vi "6060_read_all_I-O.vi"(1 "Address (Main, Sub reqd.)":T1, 2 "Channel Name":string) -> (3 "Comment":string, 4 "Input chs.":u8 format="%04b", 5 "Single Input Channel":i16)   [LabVIEW 2010]
uses:
  ADAM Client/Sub VIs/ADAM Controls/Address.ctl
panel:
  out "Output chs.":u8 format="%04b"
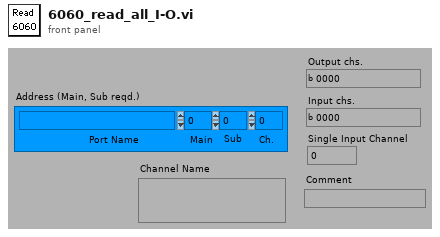
[diagram p1: front panel]
types:
  T1 = typedef "Address.ctl" = cluster{"Main":i32, "Ch.":i32, "Sub":i32, "Port Name":string}
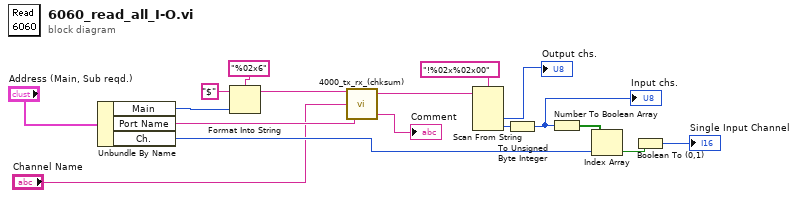
[diagram p0: block diagram]
diagram:
  n1 = Unbundle By Name("Address (Main, Sub reqd.)") -> ("Main"=w17:i32, "Port Name"=w10:string, "Ch."=w7:i32)
  n2 = Format Into String(format string="%02x6", initial string="$", w17) -> (resulting string=w14:string)  [unwired: 1 in, 1 out]
  n3 = call "4000_tx_rx_(chksum).vi"("Port Name"=w10, "Channel Name"="Channel Name", "Write String"=w14) -> ("Comment out"=→"Comment":string, "Read"=w9:string)  [unwired: 1 out]
  n4 = Scan From String(format string="!%02x%02x00", input string=w9) -> (output 1=→"Output chs.":u8, output 2=w8:i32)  [unwired: 2 in, 5 out]
  n5 = To Unsigned Byte Integer(number=w8) -> (unsigned 8bit integer=w6:u8)
  "Input chs." <- w6
  n6 = Number To Boolean Array(number=w6) -> (Boolean array=w5:bool[])
  n7 = Index Array(array=w5, index=w7) -> (element=w4:bool)
  n8 = Boolean To (0,1)(Boolean=w4) -> (0, 1=→"Single Input Channel":i16)
